vi "MecaDrivePoseEst2_Pack_Config.vi"(0 "Vision Heading std dev Rad":dbl=0.45, 3 "Front Left Wheel M":T1 {"Y" format="%14.3f"; "X" format="%14.3f"}, 4 "Vision Y std dev M":dbl=0.45, 5 "Front Right Wheel M":T1 {"Y" format="%14.3f"; "X" format="%14.3f"}, 6 "Vision X std dev M":dbl=0.45, 7 "Rear Left Wheel M":T1 {"Y" format="%14.3f"; "X" format="%14.3f"}, 8 "Odom Heading std dev Rad":dbl=0.1, 9 "Odom Y std dev M":dbl=0.1, 10 "Odom X std dev M":dbl=0.1, 11 "Rear Right Wheel M":T1 {"Y" format="%14.3f"; "X" format="%14.3f"}) -> (2 "MecaPoseEst2Config":T2={"Rear Left Wheel M"={"X"=0.0, "Y"=0.0}, "Odom X std dev M"=0.02, "Odom Y std dev M"=0.02, "Odom Heading std dev Rad"=0.01, "Vision X std dev M"=0.1, "Vision Y std dev M"=0.1, "Vision Heading std dev Rad"=0.05, "Front Left Wheel M"={"X"=0.0, "Y"=0.0}, "Front Right Wheel M"={"X"=0.0, "Y"=0.0}, "Rear Right Wheel M"={"X"=0.0, "Y"=0.0}} {"Rear Right Wheel M"."Y" format="%14.3f"; "Rear Right Wheel M"."X" format="%14.3f"; "Front Right Wheel M"."Y" format="%14.3f"; "Front Right Wheel M"."X" format="%14.3f"; "Front Left Wheel M"."Y" format="%14.3f"; "Front Left Wheel M"."X" format="%14.3f"; "Vision Heading std dev Rad" format="%#_13g"; "Vision Y std dev M" format="%#_13g"; "Vision X std dev M" format="%#_13g"; "Odom Heading std dev Rad" format="%#_13g"; "Odom Y std dev M" format="%#_13g"; "Odom X std dev M" format="%#_13g"; "Rear Left Wheel M"."Y" format="%14.3f"; "Rear Left Wheel M"."X" format="%14.3f"})   [LabVIEW 2019, in "Trajectory_Library.lvlib"]
doc: "Pack indvidual values into the cluster required by the MecaDrivePoseEst2_Execute function. \n\nInputs\n - Front Left Wheel M -- Translation2d -- Locations front left wheel in relation to center of robot. (meters)\n - Front Right Wheel M -- Translation2d -- Locations front right wheel in relation to center of robot. (meters)\n - Rear Left Wheel M -- Translation2d -- Locations rear left wheel in relation to center of robot. (meters)\n - Rear Right Wheel M -- Translation2d -- Locations rear right wheel in relation to center of robot. (meters)\n - Odom X Std Dev M -- double -- Odometry X position standard deviation (Default: 0.02) (meters)\n - Odom Y Std Dev M -- double -- Odometry Y position standard deviation (Default: 0.02) (meters)\n - Odom Heading Std Dev M -- double -- Odometry Heading (gyro) position standard deviation (Default: 0.01) (radians)\n - Vision X Std Dev M -- double -- Vision X position standard deviation (Default: 0.1) (meters)\n - Vision Y Std Dev M -- double -- Vision Y position standard deviation (Default: 0.1) (meters)\n - Vision Heading Std Dev M -- double -- Vision Heading (gyro) position standard deviation (Default: 0.05) (radians)\n\nOutputs:\n - MecaPoseEst2Config -- cluster -- Packed data values."
uses:
  Trajectory_Library.lvlib
  TypeDef/MECA_DRIVE_POSE_EST2_CONFIG.ctl
  TypeDef/TRANSLATION2D.ctl
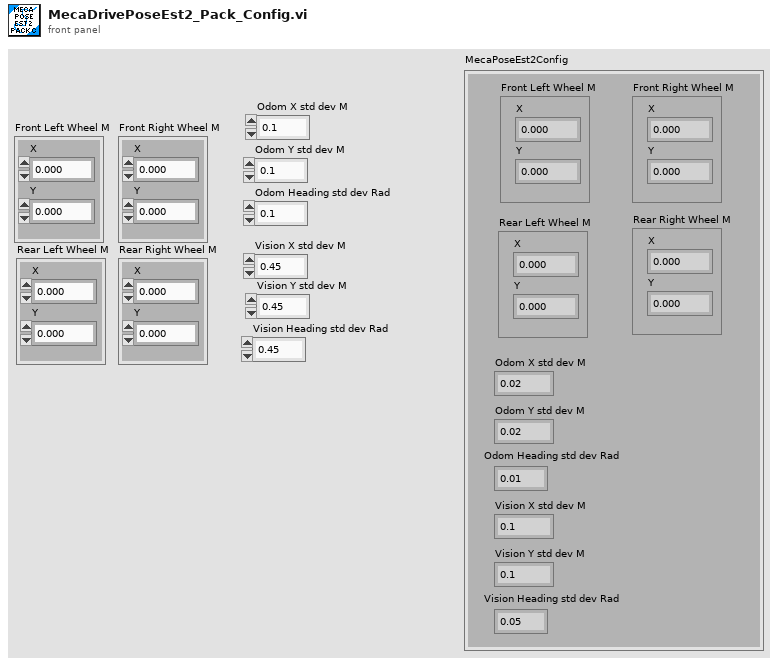
[diagram p1: front panel]
types:
  T1 = typedef "Trajectory_Library.lvlib/TRANSLATION2D.ctl" = cluster{"X":dbl, "Y":dbl}
  T2 = typedef "Trajectory_Library.lvlib/MECA_DRIVE_POSE_EST2_CONFIG.ctl" = cluster{"Rear Left Wheel M":T1, "Odom X std dev M":dbl, "Odom Y std dev M":dbl, "Odom Heading std dev Rad":dbl, "Vision X std dev M":dbl, "Vision Y std dev M":dbl, "Vision Heading std dev Rad":dbl, "Front Left Wheel M":T1, "Front Right Wheel M":T1, "Rear Right Wheel M":T1}
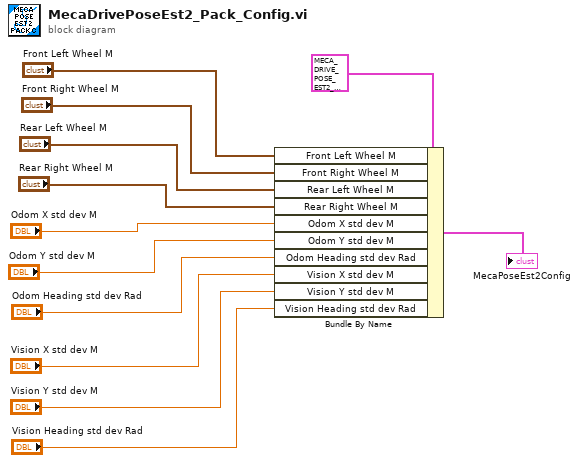
[diagram p0: block diagram]
diagram:
  n1 = Bundle By Name(cluster=T2 {"Rear Left Wheel M"={"X"=0.0, "Y"=0.0}, "Odom X std dev M"=0.02, "Odom Y std dev M"=0.02, "Odom Heading std dev Rad"=0.01, "Vision X std dev M"=0.1, "Vision Y std dev M"=0.1, "Vision Heading std dev Rad"=0.05, "Front Left Wheel M"={"X"=0.0, "Y"=0.0}, "Front Right Wheel M"={"X"=0.0, "Y"=0.0}, "Rear Right Wheel M"={"X"=0.0, "Y"=0.0}} ("MecaPoseEst2Config"), "Front Left Wheel M"="Front Left Wheel M", "Front Right Wheel M"="Front Right Wheel M", "Rear Left Wheel M"="Rear Left Wheel M", "Rear Right Wheel M"="Rear Right Wheel M", "Odom X std dev M"="Odom X std dev M", "Odom Y std dev M"="Odom Y std dev M", "Odom Heading std dev Rad"="Odom Heading std dev Rad", "Vision X std dev M"="Vision X std dev M", "Vision Y std dev M"="Vision Y std dev M", "Vision Heading std dev Rad"="Vision Heading std dev Rad") -> (→"MecaPoseEst2Config":T2)
